vi "Read Time Stamps.vi"(8 "error in (no error)":errorcluster, 11 "Loopback in":refnum<class "Loopback.lvclass">) -> (0 "error out":errorcluster, 1 "Paths":path[](array[path]), 2 "Times":timestamp[](array[timestamp]), 3 "Loopback out":refnum<class "Loopback.lvclass">)   [LabVIEW 2014, in "Loopback.lvclass"]
uses:
  Loopback.lvclass
  Loopback.lvclass/Loopback.ctl
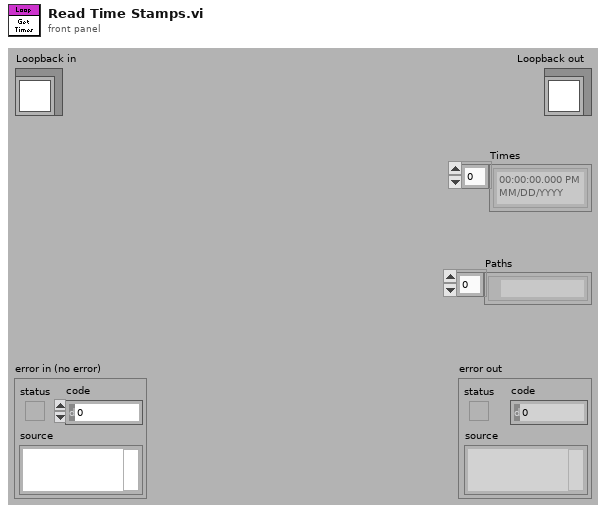
[diagram p1: front panel]
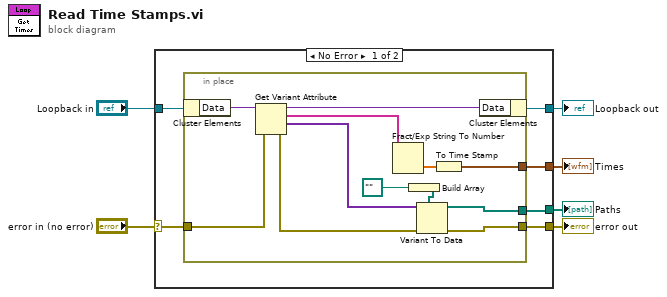
[diagram p0: block diagram]
diagram:
  n1 = case shown="No Error" "error in (no error)" {
    selector: "error in (no error)" -> [w9 w26]
    tunnel: [w8 w26] -> w5
    tunnel: [w7 w25] -> w3
    tunnel: "Loopback in" -> [w12 w25]
    tunnel: [w11 _] -> w1
    tunnel: [w10 _] -> w2
    frame No Error {
      n2 = in-place {
        in-place-border: [w15] -> w11
        in-place-border: [w18] -> w10
        in-place-border: w9 -> [w13]
        in-place-border: [w17] -> w8
        n3 = in-place-cluster #1(w12) -> ("Data"=w24:variant)
        n4 = Get Variant Attribute(Variant=w24, error in=w13) -> (duplicate Variant=w16:variant, names=w23:string[], values=w21:variant[], error out=w14:errorcluster)  [unwired: 2 in]
        n5 = Fract/Exp String To Number(string=w23) -> (number=w19:dbl[])  [unwired: 3 in, 1 out]
        n6 = Build Array(path "") -> (w20:path[])
        n7 = Variant To Data(error in=w14, type=w20, Variant=w21) -> (data=w18:path[], error out=w17:errorcluster)
        n8 = To Time Stamp(1:w19) -> (0:w15:timestamp[])
        n9 = in-place-cluster #1("Data"=w16) -> (w7:refnum<class "Loopback.lvclass">)
      }
    }
    frame Error {
    }
  }
  "error out" <- w5
  "Loopback out" <- w3
  "Paths" <- w2
  "Times" <- w1
